vi "PQfinish.vi"(8 "error in (no error)":errorcluster, 11 "conn":u64) -> (0 "error out":errorcluster)   [LabVIEW 2019, in "libpqlv64.lvlib"]
doc: "Closes the connection to the server. Also frees memory used by the PGconn object."
uses:
  libpqlv64.lvlib
  libpq.dll
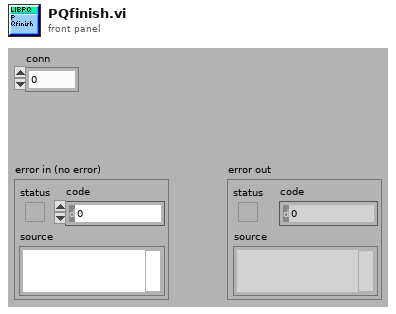
[diagram p1: front panel]
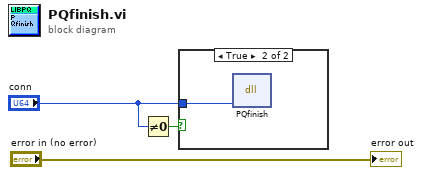
[diagram p0: block diagram]
diagram:
  n1 = Not Equal To 0?(x="conn") -> (x != 0?=w2:bool)
  n2 = case shown="True" w2 {
    tunnel: "conn" -> [_ w4]
    frame False {
    }
    frame True {
      n3 = dll-call lib="libpq.*" fn="PQfinish"("conn"=w4) -> ()  [unwired: 5 in, 2 out]
    }
  }
  "error out" <- "error in (no error)"
